vi "ReRouteAroundPolygon.vi"(2 "Desired Point Spacing (in)":dbl, 3 "AvoidancePolygon":T2, 4 "InputPath":T1[](array[typedef])) -> (0 "OutputPath":T1[](array[typedef]), 1 "PathChanged":bool)   [LabVIEW 2018, in "ArgosLib.lvlib"]
uses:
  ArgosLib.lvlib
  DeepSpaceSrc/Implements/Arm/TypeDefs/ArmAbsolutePosition.ctl
  TypeDefs/Polygon2D.ctl
  TypeDefs/Point2D.ctl
panel:
  in  "timeout(ms)":u32=1000
  out "Paths":cluster{dbl[], dbl[]}[](graph)
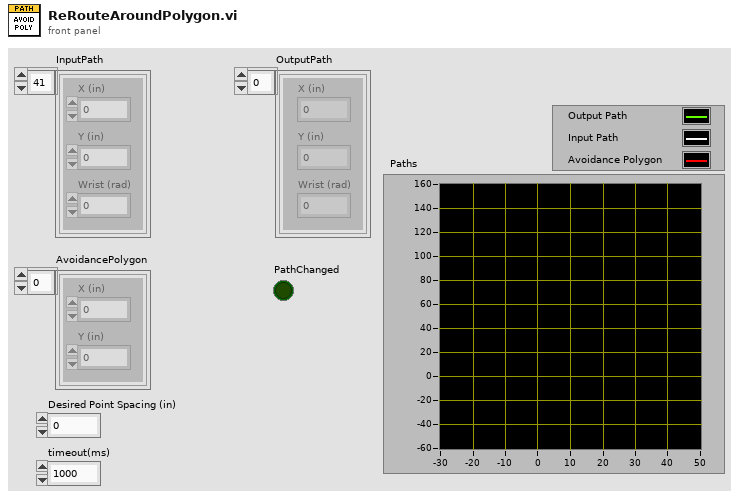
[diagram p1: front panel]
types:
  T1 = typedef "ArmAbsolutePosition.ctl" = cluster{"X (in)":dbl, "Y (in)":dbl, "Wrist (rad)":dbl}
  T2 = typedef "ArgosLib.lvlib/Polygon2D.ctl" = T3[]
  T3 = typedef "ArgosLib.lvlib/Point2D.ctl" = cluster{"X (in)":dbl, "Y (in)":dbl}
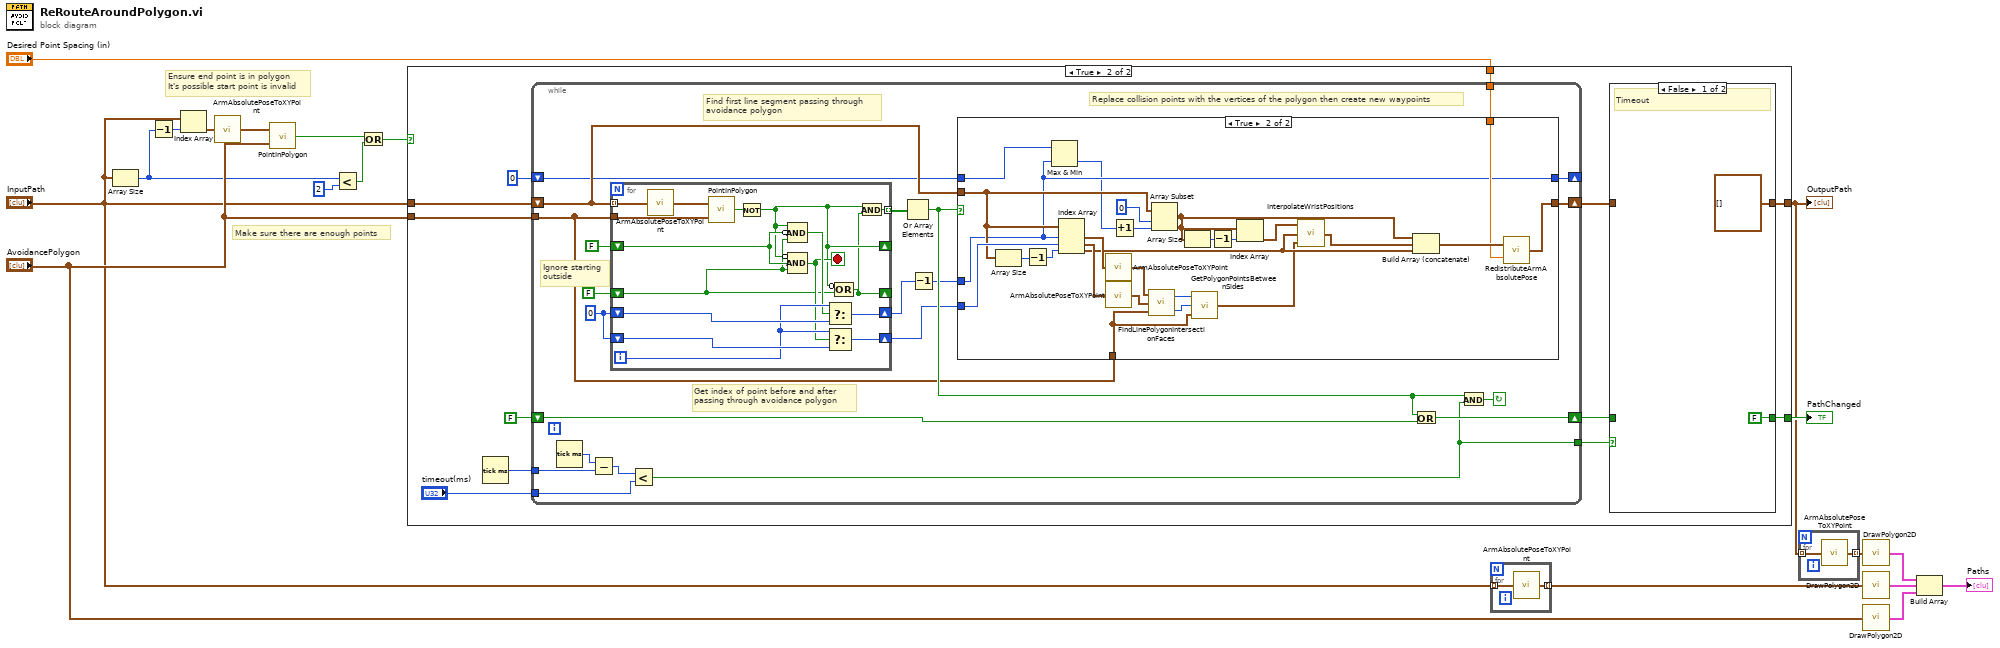
[diagram p0: block diagram]
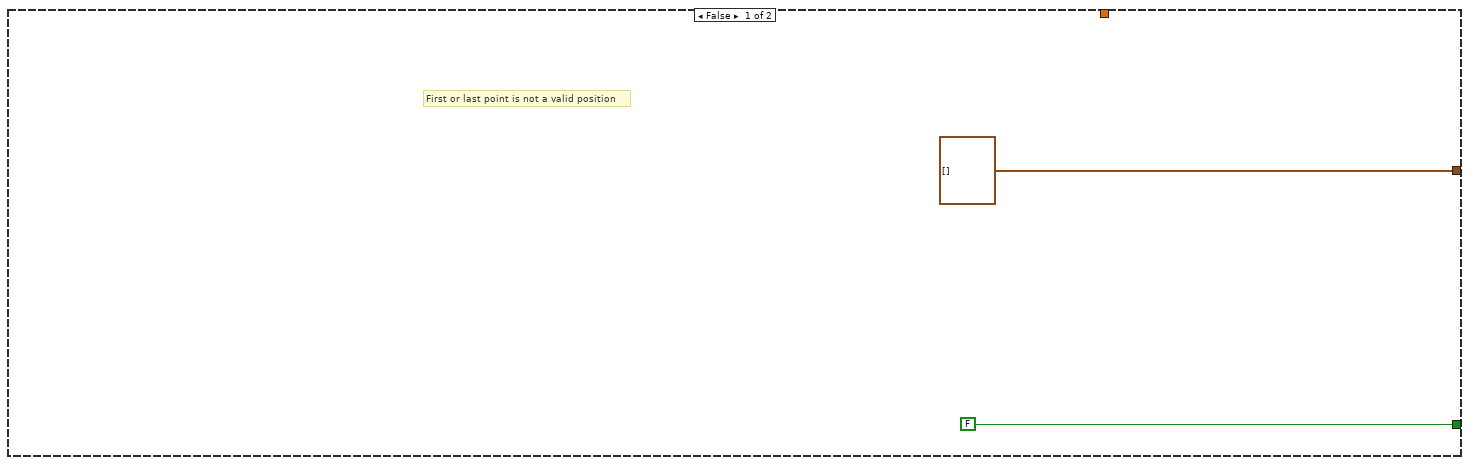
[diagram p2: hidden frame]
diagram:
  # "Ensure end point is in polygon\nIt's possible start point is invalid"
  # "Make sure there are enough points"
  n1 = Array Size(array="InputPath") -> (size(s)=w7:i32)
  n2 = Decrement(x=w7) -> (x-1=w6:i32)
  n3 = Index Array(array="InputPath", index=w6) -> (element=w8:T1)
  n4 = call "ArmAbsolutePoseToXYPoint.vi"("ArmAbsolutePose"=w8) -> ("2DPoint"=w5:T3)
  n5 = call "PointInPolygon.vi"("Polygon"="AvoidancePolygon", "2DPoint"=w5) -> ("InPolygon"=w9:bool)
  n6 = Less?(x=w7, y=2) -> (x < y?=w16:bool)
  n7 = Or(x=w9, y=w16) -> (x .or. y?=w17:bool)
  n8 = case shown="True" w17 {
    tunnel: [T1[] [] ("InputPath") w24] -> w1
    tunnel: "Desired Point Spacing (in)" -> [_ w32]
    tunnel: [FALSE w22] -> w18
    tunnel: "AvoidancePolygon" -> [_ w31]
    tunnel: "InputPath" -> [_ w30]
    frame False {
      # "First or last point is not a valid position"
    }
    frame True {
      n9 = Tick Count (ms)() -> (millisecond timer value=w28:u32)
      n10 = while {
        tunnel: w31 -> [w49]
        shift-right: [w53] -> w25
        shift-left: w30 -> [w47]
        shift-right: [w57] -> w23
        shift-left: FALSE -> [w56]
        tunnel: w32 -> [w48]
        shift-right: [w45] -> _
        shift-left: 0 -> [w44]
        tunnel: w28 -> [w43]
        tunnel: "timeout(ms)" -> [w40]
        tunnel: [w38] -> w26
        stop <- w39 continue-if-true
        w55 = 0
        # "Ignore starting\noutside"
        # "Replace collision points with the vertices of the polygon then create new waypoints"
        # "Get index of point before and after\npassing through avoidance polygon"
        # "Find first line segment passing through\navoidance polygon"
        n11 = Tick Count (ms)() -> (millisecond timer value=w42:u32)
        n12 = Subtract(x=w42, y=w43) -> (x-y=w41:u32)
        n13 = for {
          tunnel: w47 -> [w89] mode=indexing
          tunnel: w49 -> [w103]
          tunnel: [w91] -> w59 mode=indexing
          shift-right: [w92] -> _
          shift-left: FALSE -> [w102]
          shift-right: [w100] -> w52
          shift-left: w55 -> [w99]
          shift-right: [w98] -> w50
          shift-left: w55 -> [w97]
          shift-right: [w90] -> _
          shift-left: FALSE -> [w93]
          i -> [w96]
          stop <- w94 stop-if-true
          n14 = call "ArmAbsolutePoseToXYPoint.vi"("ArmAbsolutePose"=w89) -> ("2DPoint"=w88:T3)
          n15 = call "PointInPolygon.vi"("Polygon"=w103, "2DPoint"=w88) -> ("InPolygon"=w101:bool)
          n16 = Not(x=w101) -> (.not. x?=w92:bool)
          n17 = Compound Arithmetic op=AND(w92, invert w102, w93) -> (w95:bool)
          n18 = Compound Arithmetic op=AND(invert w92, w102, w93) -> (w94:bool)
          n19 = Select(t=w96, s=w95, f=w99) -> (s? t:f=w100:i32)
          n20 = Select(t=w96, s=w94, f=w97) -> (s? t:f=w98:i32)
          n21 = Compound Arithmetic op=OR(invert w92, w93) -> (w90:bool)
          n22 = And(x=w92, y=w90) -> (x .and. y?=w91:bool)
        }
        n23 = Less?(x=w41, y=w40) -> (x < y?=w38:bool)
        n24 = Or Array Elements(Boolean array=w59) -> (logical OR=w54:bool)
        n25 = Decrement(x=w52) -> (x-1=w51:i32)
        n26 = case shown="True" w54 {
          tunnel: w47 -> [w61 w81]
          tunnel: [w61 w78] -> w53
          tunnel: w51 -> [_ w63]
          tunnel: w50 -> [_ w87]
          tunnel: w49 -> [_ w84]
          tunnel: w48 -> [_ w65]
          tunnel: [w60 w63] -> w45
          tunnel: w44 -> [w60 w64]
          frame False {
            # "Path no longer goes through avoidance polygon"
          }
          frame True {
            n27 = Array Size(array=w81) -> (size(s)=w83:i32)
            n28 = Decrement(x=w83) -> (x-1=w82:i32)
            n29 = Max & Min(x=w64, y=w63) -> (min(x,y)=w62:i32)  [unwired: 1 out]
            n30 = Index Array(array=w81, index #1=w63, index #2=w87, index #3=w82) -> (element #1=w77:T1, element #2=w75:T1, element #3=w69:T1)
            n31 = call "ArmAbsolutePoseToXYPoint.vi"("ArmAbsolutePose"=w77) -> ("2DPoint"=w76:T3)
            n32 = call "ArmAbsolutePoseToXYPoint.vi"("ArmAbsolutePose"=w75) -> ("2DPoint"=w74:T3)
            n33 = Increment(x=w62) -> (x+1=w79:i32)
            n34 = call "FindLinePolygonIntersectionFaces.vi"("Polygon"=w84, "ExitPoint"=w74, "EntryPoint"=w76) -> ("Exit Face"=w85:i32, "Entry Face"=w86:i32)
            n35 = Array Subset(array=w81, index=0, length=w79) -> (w72:T1[])
            n36 = Array Size(array=w72) -> (size(s)=w73:i32)
            n37 = call "GetPolygonPointsBetweenSides.vi"("Polygon"=w84, "LastSideIndex"=w85, "FirstSideIndex"=w86) -> ("PolygonVertices"=w68:T3[])
            n38 = Decrement(x=w73) -> (x-1=w71:i32)
            n39 = Index Array(array=w72, index=w71) -> (element=w70:T1)
            n40 = call "InterpolateWristPositions.vi"("MiddlePoints"=w68, "SubsequentPose"=w69, "PriorPose"=w70) -> ("ConvertedPoints"=w67:T1[])
            n41 = Build Array (concatenate)(w72, w67, w69) -> (w66:T1[])
            n42 = call "RedistributeArmAbsolutePose.vi"("DesiredPointSpacing (in)"=w65, "OriginalPoints"=w66) -> ("RedistributedPoints"=w78:T1[])
          }
        }
        n43 = Or(x=w54, y=w56) -> (x .or. y?=w57:bool)
        n44 = And(x=w54, y=w38) -> (x .and. y?=w39:bool)
      }
      n45 = case shown="False" w26 {
        tunnel: w25 -> [_ w37]
        tunnel: [T1[] [] ("InputPath") w37] -> w24
        tunnel: w23 -> [_ w36]
        tunnel: [FALSE w36] -> w22
        frame False {
          # "Timeout"
        }
        frame True {
          # "No Timeout"
        }
      }
    }
  }
  "OutputPath" <- w1
  "PathChanged" <- w18
  n46 = for {
    tunnel: "InputPath" -> [w105] mode=indexing
    tunnel: [w104] -> w3 mode=indexing
    n47 = call "ArmAbsolutePoseToXYPoint.vi"("ArmAbsolutePose"=w105) -> ("2DPoint"=w104:T3)
  }
  n48 = for {
    tunnel: w1 -> [w107] mode=indexing
    tunnel: [w106] -> w2 mode=indexing
    n49 = call "ArmAbsolutePoseToXYPoint.vi"("ArmAbsolutePose"=w107) -> ("2DPoint"=w106:T3)
  }
  n50 = call "DrawPolygon2D.vi"("Polygon"=w2) -> ("XYPlot"=w13:cluster{dbl[], dbl[]})
  n51 = call "DrawPolygon2D.vi"("Polygon"=w3) -> ("XYPlot"=w12:cluster{dbl[], dbl[]})
  n52 = call "DrawPolygon2D.vi"("Polygon"="AvoidancePolygon") -> ("XYPlot"=w11:cluster{dbl[], dbl[]})
  n53 = Build Array(w13, w12, w11) -> (→"Paths":cluster{dbl[], dbl[]}[])
